vi "Read_Gas_Desk_file.vi"(0 "File string In":string, 1 "Filename":path) -> (2 "Channel names":string[](array[string]), 3 "Valid File?":bool, 4 "Ch Values":string[][](table))   [LabVIEW 2010]
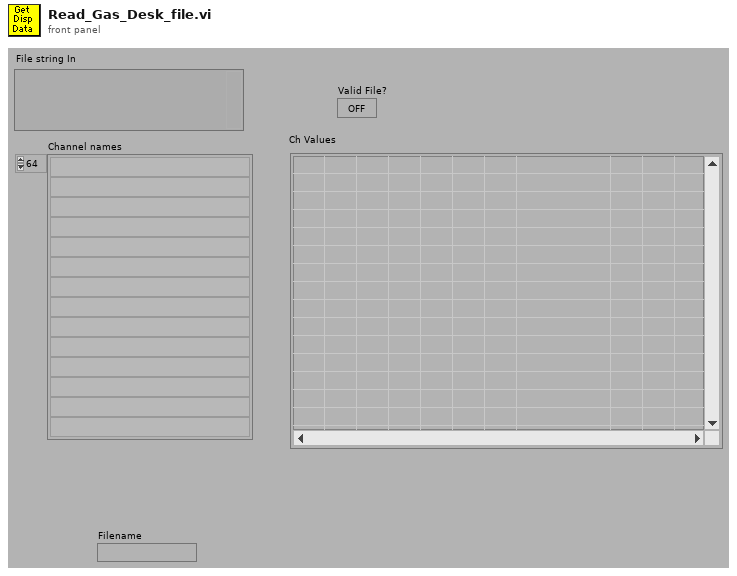
[diagram p1: front panel]
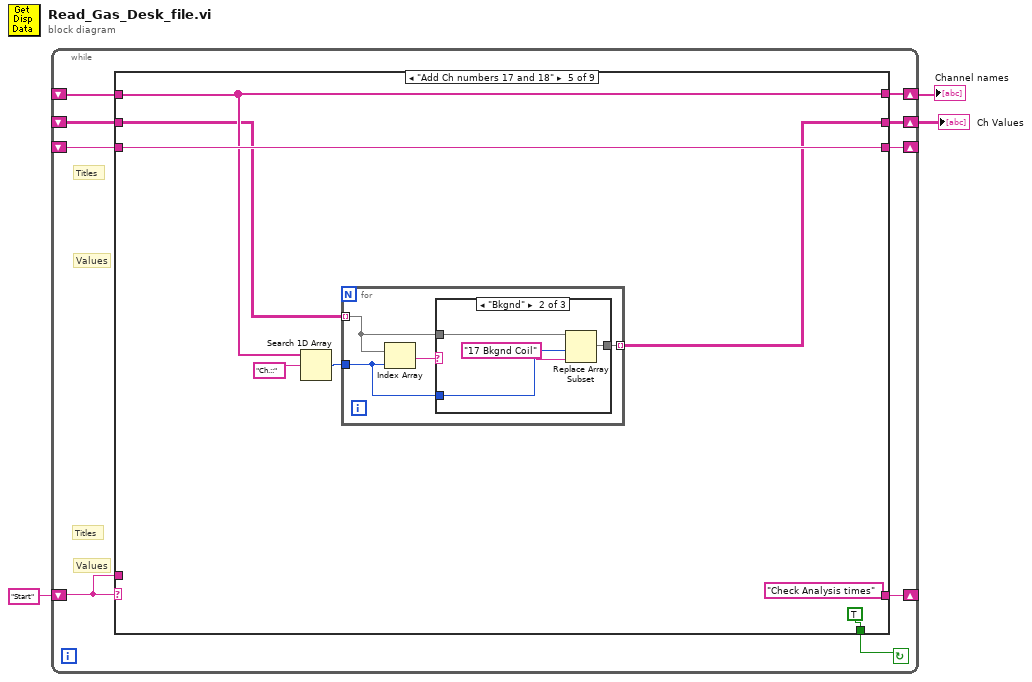
[diagram p0: block diagram]
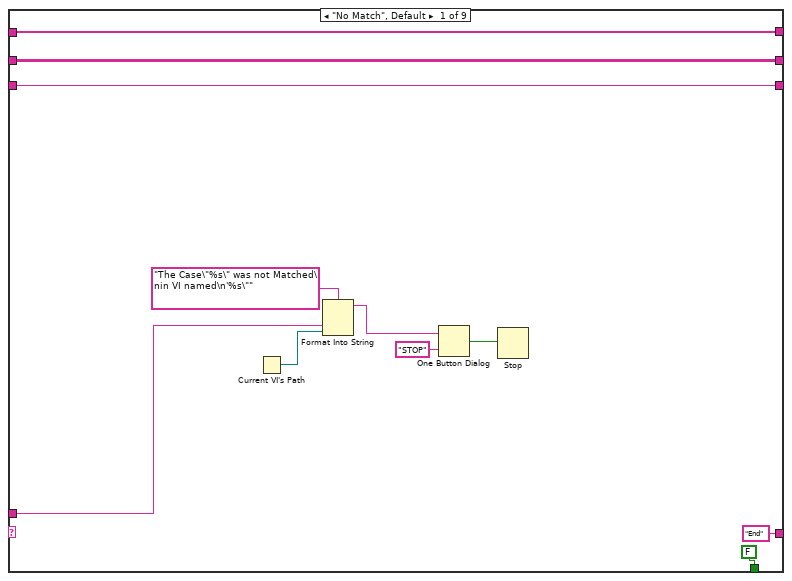
[diagram p2: hidden frame]
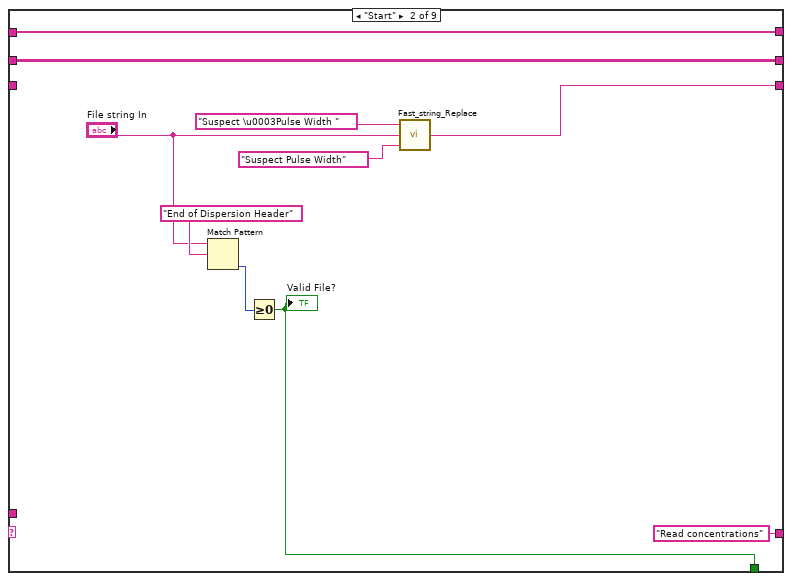
[diagram p3: hidden frame]
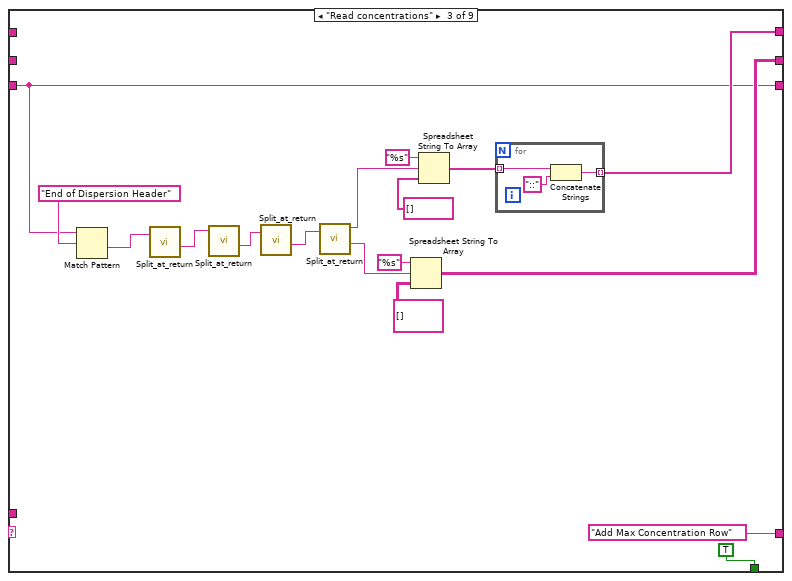
[diagram p4: hidden frame]
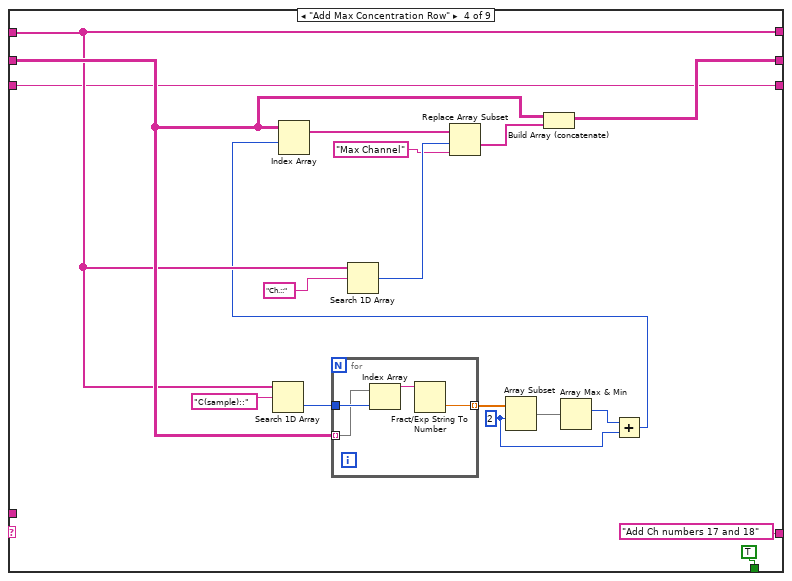
[diagram p5: hidden frame]
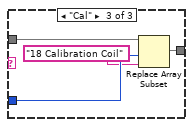
[diagram p7: hidden frame]
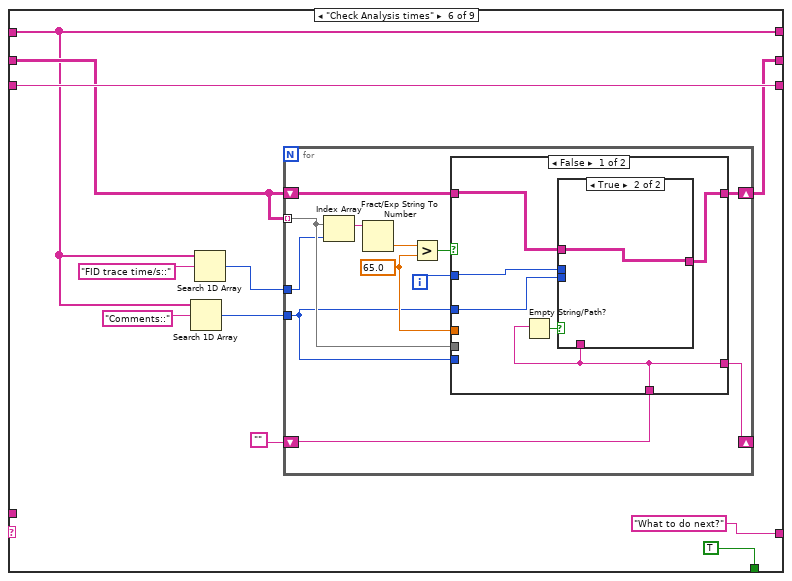
[diagram p8: hidden frame]
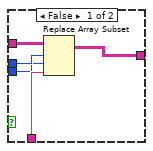
[diagram p9: hidden frame]
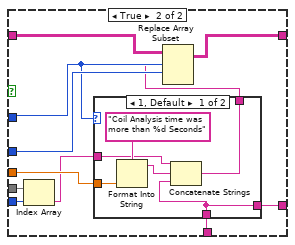
[diagram p10: hidden frame]
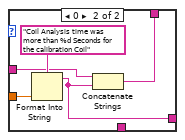
[diagram p11: hidden frame]
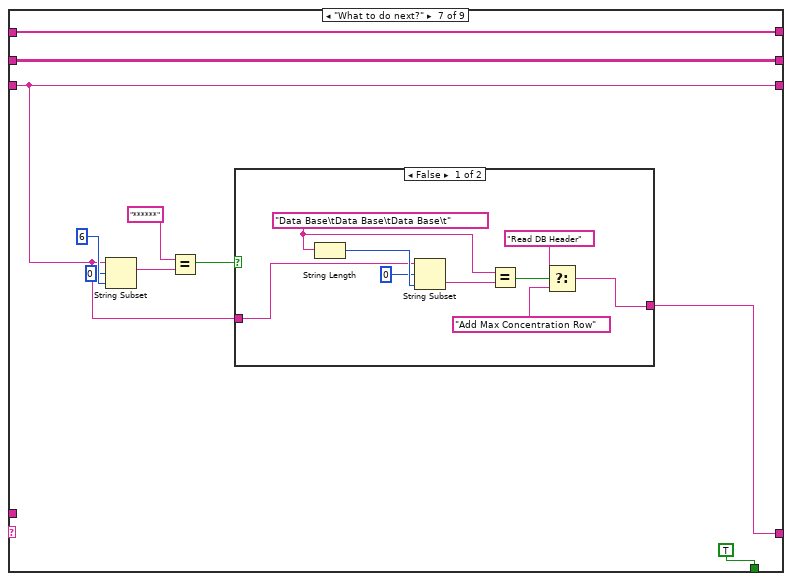
[diagram p12: hidden frame]
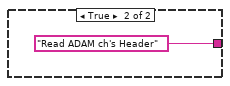
[diagram p13: hidden frame]
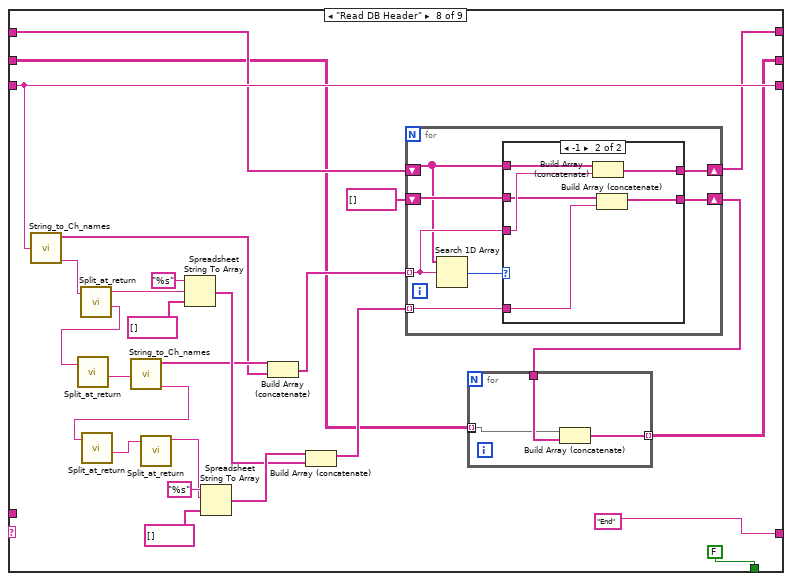
[diagram p14: hidden frame]
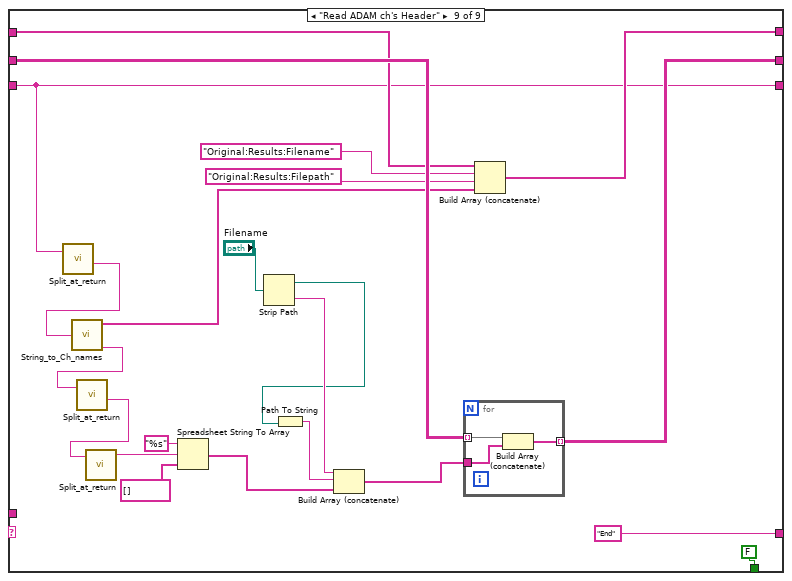
[diagram p16: hidden frame]
diagram:
  n1 = while {
    shift-left: _ -> [w6]
    shift-right: [w7] -> _
    shift-left: _ -> [w8]
    shift-right: [w10] -> w1
    shift-left: _ -> [w9]
    shift-right: [w11] -> w2
    shift-left: "Start" -> [w12]
    shift-right: [w5] -> _
    stop <- w4 continue-if-true
    # "Values"
    # "Titles"
    # "Values"
    # "Titles"
    n2 = case shown="\"Add Ch numbers 17 and 18\"" w12 {
      tunnel: w12 -> [w18 _ _ _ _ _ _ _ _]
      tunnel: [w15 w31 w37 w62 w79 w97 w154 w177 w236] -> w11
      tunnel: [w16 w30 w36 w63 w76 w102 w155 w174 w237] -> w10
      tunnel: w9 -> [w15 w31 _ w62 w79 w97 w154 w180 w238]
      tunnel: w8 -> [w16 w30 _ w64 w78 w98 w155 w176 w239]
      tunnel: [w17 w26 w35 w61 w82 w103 w156 w196 w235] -> w7
      tunnel: w6 -> [w17 _ w35 w61 w82 w103 w156 w196 w235]
      tunnel: ["End" "Read concentrations" "Add Max Concentration Row" "Add Ch numbers 17 and 18" "Check Analysis times" "What to do next?" w157 "End" "End"] -> w5
      tunnel: [FALSE w24 TRUE TRUE TRUE TRUE TRUE FALSE FALSE] -> w4
      frame "No Match", Default {
        n3 = Current VI's Path() -> (path=w19:path)
        n4 = Format Into String(format string="The Case\"%s\" was not Matched\nin VI named\n'%s\"" ("Format String"), w18, w19) -> (resulting string=w22:string)  [unwired: 2 in, 1 out]
        n5 = One Button Dialog(message=w22, button name ("OK")="STOP") -> (true=w20:bool)
        n6 = Stop(stop? (T)=w20) -> ()
      }
      frame "Start" {
        n7 = Match Pattern(string="File string In", regular expression="End of Dispersion Header") -> (offset past match=w32:i32)  [unwired: 1 in, 3 out]
        n8 = Greater Or Equal To 0?(x=w32) -> (x >= 0?=w24:bool)
        "Valid File?" <- w24
        n9 = call "Fast_string_Replace.vi"("Replace match with:"="Suspect Pulse Width" ("regular expression"), "Input String"="File string In", "regular expression"="Suspect \u0003Pulse Width ") -> ("Output String"=w26:string)  [unwired: 1 in, 1 out]
      }
      frame "Read concentrations" {
        n10 = Match Pattern(string=w35, regular expression="End of Dispersion Header") -> (after substring=w49:string)  [unwired: 1 in, 3 out]
        n11 = call "Split_at_return.vi"("String"=w49) -> ("after substring"=w48:string)  [unwired: 1 in, 3 out]
        n12 = call "Split_at_return.vi"("String"=w48) -> ("after substring"=w47:string)  [unwired: 1 in, 3 out]
        n13 = call "Split_at_return.vi"("String"=w47) -> ("after substring"=w46:string)  [unwired: 1 in, 3 out]
        n14 = call "Split_at_return.vi"("String"=w46) -> ("before substring"=w43:string, "after substring"=w40:string)  [unwired: 1 in, 2 out]
        n15 = Spreadsheet String To Array(format string="%s", spreadsheet string=w40, array type (2D Dbl)=string[][] [] ("Output Array")) -> (array=w36:string[][])  [unwired: 1 in]
        n16 = Spreadsheet String To Array(format string="%s", spreadsheet string=w43, array type (2D Dbl)=string[] [] ("Output Array")) -> (array=w39:string[])  [unwired: 1 in]
        n17 = for {
          tunnel: [w52] -> w37 mode=indexing
          tunnel: w39 -> [w51] mode=indexing
          n18 = Concatenate Strings(w51, "::" ("Substring")) -> (w52:string)
        }
      }
      frame "Add Max Concentration Row" {
        w55 = 2 ("Array Index")
        n19 = Search 1D Array(1D array=w62, element="C(sample)::") -> (index of element=w70:i32)  [unwired: 1 in]
        n20 = for {
          tunnel: w64 -> [w73] mode=indexing
          tunnel: w70 -> [w75]
          tunnel: [w72] -> w58 mode=indexing
          n21 = Index Array(array=w73, index=w75) -> (element=w74:string)
          n22 = Fract/Exp String To Number(string=w74) -> (number=w72:dbl)  [unwired: 3 in, 1 out]
        }
        n23 = Search 1D Array(1D array=w62, element="Ch.::") -> (index of element=w68:i32)  [unwired: 1 in]
        n24 = Array Subset(array=w58, index=w55) -> (w57:dbl[])  [unwired: 1 in]
        n25 = Array Max & Min(array=w57) -> (max index (indices)=w56:i32)  [unwired: 3 out]
        n26 = Add(x=w56, y=w55) -> (x+y=w54:i32)
        n27 = Index Array(array=w64, index (row)=w54) -> (element=w67:string[])  [unwired: 1 in]
        n28 = Replace Array Subset(array=w67, new element="Max Channel" ("Element Data"), index=w68) -> (w65:string[])
        n29 = Build Array (concatenate)(w64, w65) -> (w63:string[][])
      }
      frame "Add Ch numbers 17 and 18" {
        n30 = Search 1D Array(1D array=w79, element="Ch.::") -> (index of element=w77:i32)  [unwired: 1 in]
        n31 = for {
          tunnel: w78 -> [w84] mode=indexing
          tunnel: w77 -> [w85]
          tunnel: [w86] -> w76 mode=indexing
          n32 = Index Array(array=w84, index=w85) -> (element=w87:string)
          n33 = case shown="\"Bkgnd\"" w87 {
            tunnel: [w88 w90 w94] -> w86
            tunnel: w85 -> [_ w92 w96]
            tunnel: w84 -> [w88 w91 w95]
            frame "No Match", Default {
            }
            frame "Bkgnd" {
              n34 = Replace Array Subset(array=w91, new element="17 Bkgnd Coil", index=w92) -> (w90:string[])
            }
            frame "Cal" {
              n35 = Replace Array Subset(array=w95, new element="18 Calibration Coil", index=w96) -> (w94:string[])
            }
          }
        }
      }
      frame "Check Analysis times" {
        n36 = Search 1D Array(1D array=w97, element="Comments::") -> (index of element=w104:i32)  [unwired: 1 in]
        n37 = Search 1D Array(1D array=w97, element="FID trace time/s::") -> (index of element=w105:i32)  [unwired: 1 in]
        n38 = for {
          tunnel: w105 -> [w109]
          shift-right: [w118] -> w102
          shift-left: w98 -> [w116]
          tunnel: w104 -> [w108]
          shift-right: [w115] -> _
          shift-left: "" -> [w114]
          tunnel: w98 -> [w110] mode=indexing
          i -> [w111]
          w112 = 65.0 ("y")
          n39 = Index Array(array=w110, index=w109) -> (element=w113:string)
          n40 = Fract/Exp String To Number(string=w113) -> (number=w119:dbl)  [unwired: 3 in, 1 out]
          n41 = Greater?(x=w119, y=w112) -> (0:w117:bool)
          n42 = case shown="False" w117 {
            tunnel: w111 -> [w121 w139]
            tunnel: w108 -> [w120 w140]
            tunnel: w116 -> [w124 w142]
            tunnel: [w123 w141] -> w118
            tunnel: [w122 w137] -> w115
            tunnel: w114 -> [w122 w138]
            tunnel: w112 -> [_ w135]
            tunnel: w110 -> [_ w134]
            tunnel: w108 -> [_ w133]
            frame False {
              n43 = Empty String/Path?(string/path=w122) -> (empty?=w125:bool)
              n44 = case shown="True" w125 {
                tunnel: w124 -> [w130 w131]
                tunnel: [w129 w131] -> w123
                tunnel: w122 -> [w128 _]
                tunnel: w121 -> [w127 _]
                tunnel: w120 -> [w126 _]
                frame False {
                  n45 = Replace Array Subset(array=w130, new element=w128, index (row)=w127, index (col)=w126) -> (w129:string[][])
                }
                frame True {
                }
              }
            }
            frame True {
              n46 = Index Array(array=w134, index=w133) -> (element=w132:string)
              n47 = case shown="1, Default" w139 {
                tunnel: w135 -> [w147 w153]
                tunnel: w132 -> [w145 w151]
                tunnel: w138 -> [w144 _]
                tunnel: [w144 w149] -> w137
                tunnel: [w143 w150] -> w136
                frame 1, Default {
                  n48 = Format Into String(format string="Coil Analysis time was more than %d Seconds", w147) -> (resulting string=w148:string)  [unwired: 2 in, 1 out]
                  n49 = Concatenate Strings(w145, w148, w144) -> (w143:string)
                }
                frame 0 {
                  n50 = Format Into String(format string="Coil Analysis time was more than %d Seconds for the calibration Coil", w153) -> (resulting string=w149:string)  [unwired: 2 in, 1 out]
                  n51 = Concatenate Strings(w151, w149) -> (w150:string)
                }
              }
              n52 = Replace Array Subset(array=w142, new element=w136, index (row)=w139, index (col)=w140) -> (w141:string[][])
            }
          }
        }
      }
      frame "What to do next?" {
        n53 = String Subset(string=w156, offset (0)=0, length (rest)=6 ("length")) -> (substring=w161:string)
        n54 = Equal?(x="******", y=w161) -> (x = y?=w159:bool)
        n55 = case shown="False" w159 {
          tunnel: [w165 "Read ADAM ch's Header"] -> w157
          tunnel: w156 -> [w164 _]
          frame False {
            w169 = "Data Base\tData Base\tData Base\t"
            n56 = String Length(string=w169) -> (length=w172:i32)
            n57 = String Subset(string=w164, offset (0)=0, length (rest)=w172) -> (substring=w170:string)
            n58 = Equal?(x=w169, y=w170) -> (x = y?=w168:bool)
            n59 = Select(t="Read DB Header", s=w168, f="Add Max Concentration Row") -> (s? t:f=w165:string)
          }
          frame True {
          }
        }
      }
      frame "Read DB Header" {
        n60 = call "String_to_Ch_names.vi"("Spreadsheet string"=w196) -> ("Ch names"=w181:string[], "String After names"=w197:string)  [unwired: 2 out]
        n61 = call "Split_at_return.vi"("String"=w197) -> ("before substring"=w193:string, "after substring"=w192:string)  [unwired: 1 in, 2 out]
        n62 = call "Split_at_return.vi"("String"=w192) -> ("after substring"=w191:string)  [unwired: 1 in, 3 out]
        n63 = call "String_to_Ch_names.vi"("Spreadsheet string"=w191) -> ("Ch names"=w182:string[], "String After names"=w190:string)  [unwired: 2 out]
        n64 = call "Split_at_return.vi"("String"=w190) -> ("after substring"=w187:string)  [unwired: 1 in, 3 out]
        n65 = call "Split_at_return.vi"("String"=w187) -> ("before substring"=w186:string)  [unwired: 1 in, 3 out]
        n66 = Spreadsheet String To Array(format string="%s", spreadsheet string=w193, array type (2D Dbl)=string[] [] ("Channel Values")) -> (array=w183:string[])  [unwired: 1 in]
        n67 = Spreadsheet String To Array(format string="%s", spreadsheet string=w186, array type (2D Dbl)=string[] [] ("Channel Values")) -> (array=w184:string[])  [unwired: 1 in]
        n68 = Build Array (concatenate)(w182, w181) -> (w179:string[])
        n69 = Build Array (concatenate)(w184, w183) -> (w178:string[])
        n70 = for {
          tunnel: w179 -> [w207] mode=indexing
          shift-right: [w205] -> w175
          shift-left: string[] [] -> [w206]
          shift-right: [w208] -> w177
          shift-left: w180 -> [w203]
          tunnel: w178 -> [w204] mode=indexing
          n71 = Search 1D Array(1D array=w203, element=w207) -> (index of element=w209:i32)  [unwired: 1 in]
          n72 = case shown="-1" w209 {
            tunnel: w203 -> [w211 w217]
            tunnel: [w211 w216] -> w208
            tunnel: w207 -> [_ w215]
            tunnel: w206 -> [w210 w214]
            tunnel: [w210 w213] -> w205
            tunnel: w204 -> [_ w212]
            frame 0, Default {
            }
            frame -1 {
              n73 = Build Array (concatenate)(w217, w215) -> (w216:string[])
              n74 = Build Array (concatenate)(w214, w212) -> (w213:string[])
            }
          }
        }
        n75 = for {
          tunnel: [w200] -> _ mode=indexing
          tunnel: w175 -> [w202]
          tunnel: [w201] -> w174 mode=indexing
          tunnel: w176 -> [w200] mode=indexing
          n76 = Build Array (concatenate)(w200, w202) -> (w201:string[])
        }
      }
      frame "Read ADAM ch's Header" {
        n77 = call "Split_at_return.vi"("String"=w235) -> ("after substring"=w223:string)  [unwired: 1 in, 3 out]
        n78 = call "String_to_Ch_names.vi"("Spreadsheet string"=w223) -> ("Ch names"=w220:string[], "String After names"=w222:string)  [unwired: 2 out]
        n79 = call "Split_at_return.vi"("String"=w222) -> ("after substring"=w221:string)  [unwired: 1 in, 3 out]
        n80 = call "Split_at_return.vi"("String"=w221) -> ("before substring"=w224:string)  [unwired: 1 in, 3 out]
        n81 = Spreadsheet String To Array(format string="%s", spreadsheet string=w224, array type (2D Dbl)=string[] [] ("Channel Values")) -> (array=w219:string[])  [unwired: 1 in]
        n82 = Strip Path(path="Filename") -> (stripped path=w230:path, name=w231:string)
        n83 = Path To String(path=w230) -> (string=w229:string)
        n84 = Build Array (concatenate)(w231, w229, w219) -> (w232:string[])
        n85 = for {
          tunnel: [w242] -> w237 mode=indexing
          tunnel: w232 -> [w241]
          tunnel: w239 -> [w240] mode=indexing
          n86 = Build Array (concatenate)(w240, w241) -> (w242:string[])
        }
        n87 = Build Array (concatenate)(w238, "Original:Results:Filename", "Original:Results:Filepath", w220) -> (w236:string[])
      }
    }
  }
  "Channel names" <- w2
  "Ch Values" <- w1
